vi "test Format RESP3.vi"() -> (0 "error out":errorcluster, 2 "pass?":bool)   [LabVIEW 2019, in "RESP3 Tests.lvlib"]
uses:
  RESP3 Tests.lvlib
  RESP3/RESP3 Parser/RESP3 Parser.lvclass
  RESP3/types/RESP3 data type attribute.vi
  RESP3/high-level/RESP3 Make Simple String.vi
  RESP3/high-level/RESP3 Make Simple Error.vi
  RESP3/high-level/RESP3 Make Bulk String.vi
  RESP3/high-level/RESP3 Make Bulk Error.vi
  RESP3/high-level/RESP3 Make Map.vi
  RESP3/high-level/RESP3 Make Attributes.vi
  RESP3/high-level/RESP3 Make Set.vi
  RESP3/high-level/RESP3 Make Array.vi
  RESP3/RESP3.lvlib
panel:
  out "values match?":bool
  out "RESP3 Value orig.":variant
  out "RESP3 Value reparsed":variant
  out "messages":string[](array[string])
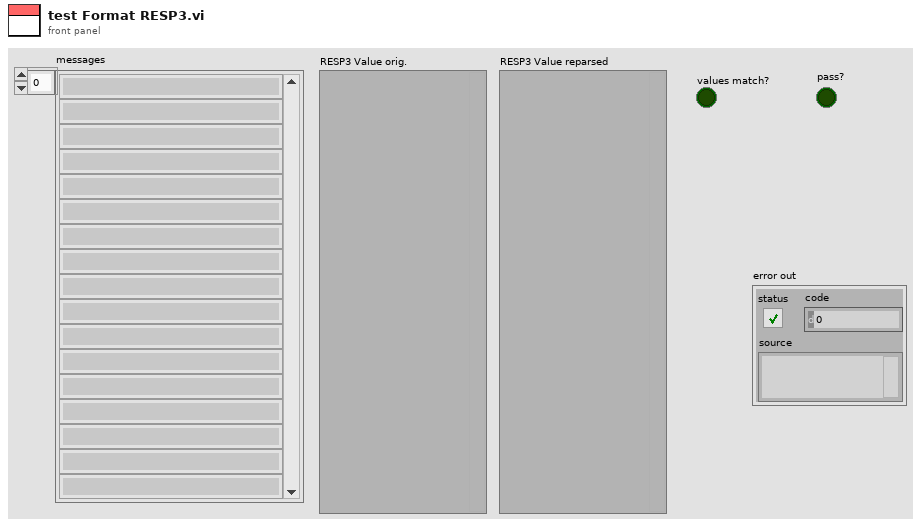
[diagram p1: front panel]
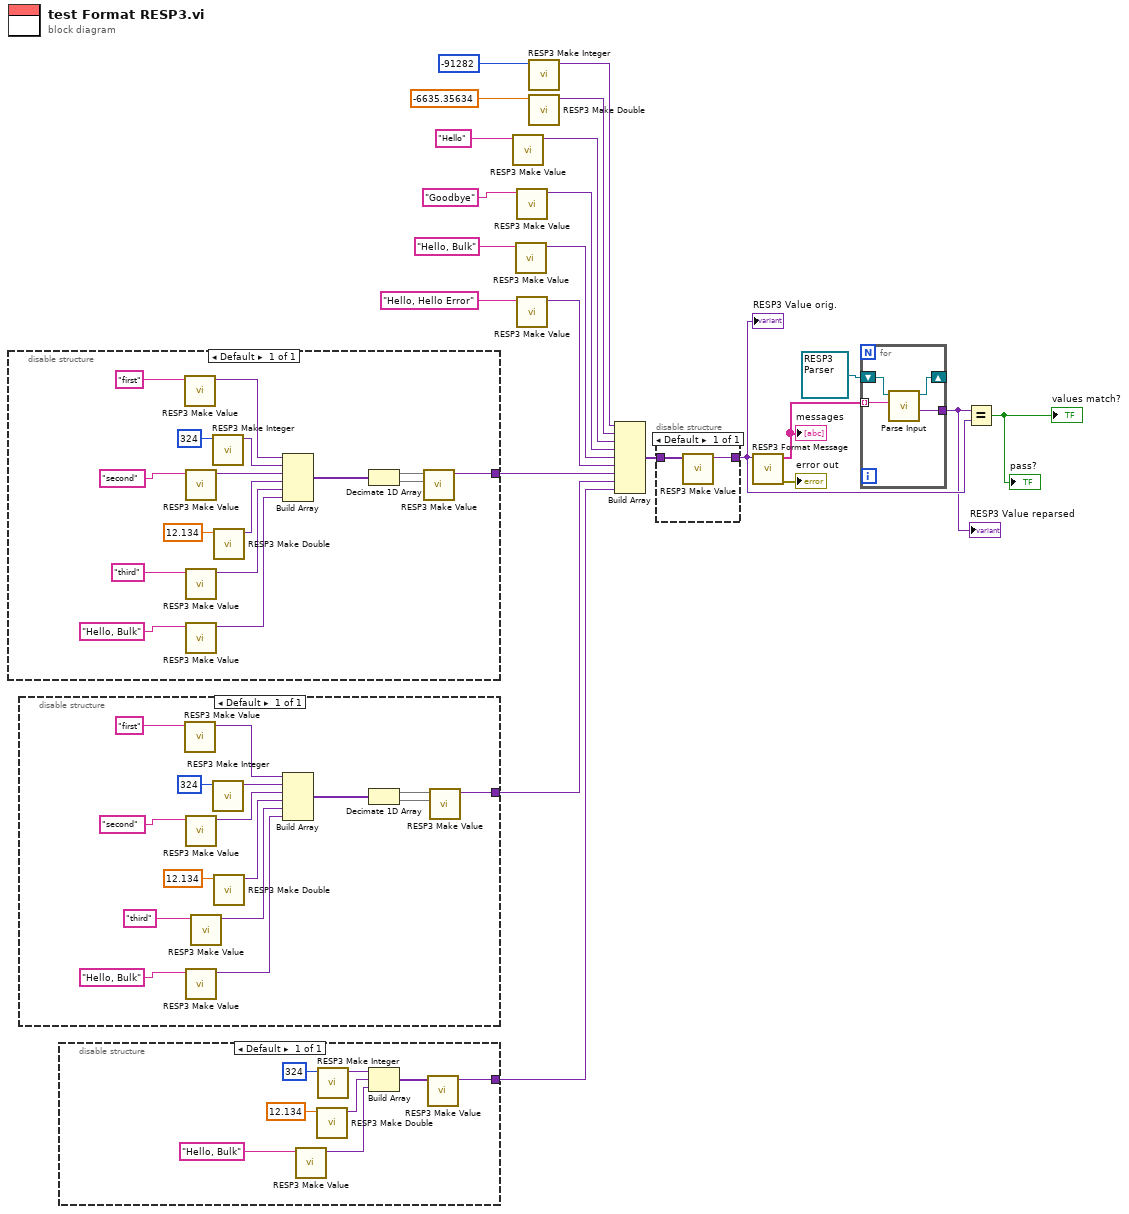
[diagram p0: block diagram]
diagram:
  n1 = disable-structure shown="Default" {
    disable-tunnel: [w26] -> w12
    frame Enabled {
      n2 = call-poly "RESP3 Make Value.vi"("String"="first" ("string in")) -> ("RESP3 Value out"=w37:variant)  [unwired: 9 in, 1 out]
      n3 = call-poly "RESP3 Make Value.vi"("String"="second" ("string in")) -> ("RESP3 Value out"=w35:variant)  [unwired: 9 in, 1 out]
      n4 = call-poly "RESP3 Make Value.vi"("String"="third" ("string in")) -> ("RESP3 Value out"=w33:variant)  [unwired: 9 in, 1 out]
      n5 = call-poly "RESP3 Make Value.vi"("String"="Hello, Bulk" ("string in")) -> ("RESP3 Value out"=w32:variant)  [unwired: 9 in, 1 out]
      n6 = call "RESP3 Make Integer.vi"("integer"=i64 324) -> ("RESP3 Value out"=w36:variant)  [unwired: 9 in, 1 out]
      n7 = call "RESP3 Make Double.vi"("double"=12.134) -> ("RESP3 Value out"=w34:variant)  [unwired: 9 in, 1 out]
      n8 = Build Array(w37, w36, w35, w34, w33, w32) -> (w25:variant[])
      n9 = Decimate 1D Array(w25) -> (w24:variant[], w23:variant[])
      n10 = call-poly "RESP3 Make Value.vi"("values (RESP3 values)"=w23, "keys (RESP3 values)"=w24) -> ("RESP3 Value out"=w26:variant)  [unwired: 8 in, 1 out]
    }
  }
  n11 = disable-structure shown="Default" {
    disable-tunnel: [w42] -> w5
    frame Enabled {
      n12 = call-poly "RESP3 Make Value.vi"("String"="first" ("string in")) -> ("RESP3 Value out"=w52:variant)  [unwired: 9 in, 1 out]
      n13 = call-poly "RESP3 Make Value.vi"("String"="second" ("string in")) -> ("RESP3 Value out"=w50:variant)  [unwired: 9 in, 1 out]
      n14 = call-poly "RESP3 Make Value.vi"("String"="Hello, Bulk" ("string in")) -> ("RESP3 Value out"=w47:variant)  [unwired: 9 in, 1 out]
      n15 = call-poly "RESP3 Make Value.vi"("String"="third" ("string in")) -> ("RESP3 Value out"=w48:variant)  [unwired: 9 in, 1 out]
      n16 = call "RESP3 Make Integer.vi"("integer"=i64 324) -> ("RESP3 Value out"=w51:variant)  [unwired: 9 in, 1 out]
      n17 = call "RESP3 Make Double.vi"("double"=12.134) -> ("RESP3 Value out"=w49:variant)  [unwired: 9 in, 1 out]
      n18 = Build Array(w52, w51, w50, w49, w48, w47) -> (w41:variant[])
      n19 = Decimate 1D Array(w41) -> (w40:variant[], w39:variant[])
      n20 = call-poly "RESP3 Make Value.vi"("values (RESP3 values)"=w39, "keys (RESP3 values)"=w40) -> ("RESP3 Value out"=w42:variant)  [unwired: 8 in, 1 out]
    }
  }
  n21 = disable-structure shown="Default" {
    disable-tunnel: [w56] -> w4
    frame Enabled {
      n22 = call-poly "RESP3 Make Value.vi"("String"="Hello, Bulk" ("string in")) -> ("RESP3 Value out"=w58:variant)  [unwired: 9 in, 1 out]
      n23 = call "RESP3 Make Double.vi"("double"=12.134) -> ("RESP3 Value out"=w59:variant)  [unwired: 9 in, 1 out]
      n24 = call "RESP3 Make Integer.vi"("integer"=i64 324) -> ("RESP3 Value out"=w60:variant)  [unwired: 9 in, 1 out]
      n25 = Build Array(w60, w59, w58) -> (w55:variant[])
      n26 = call-poly "RESP3 Make Value.vi"("RESP3 Values in"=w55) -> ("RESP3 Value out"=w56:variant)  [unwired: 9 in, 1 out]
    }
  }
  n27 = call-poly "RESP3 Make Value.vi"("String"="Hello" ("string in")) -> ("RESP3 Value out"=w17:variant)  [unwired: 9 in, 1 out]
  n28 = call-poly "RESP3 Make Value.vi"("String"="Hello, Bulk" ("string in")) -> ("RESP3 Value out"=w15:variant)  [unwired: 9 in, 1 out]
  n29 = call-poly "RESP3 Make Value.vi"("String"="Goodbye" ("string in")) -> ("RESP3 Value out"=w16:variant)  [unwired: 9 in, 1 out]
  n30 = call-poly "RESP3 Make Value.vi"("String"="Hello, Hello Error" ("string in")) -> ("RESP3 Value out"=w14:variant)  [unwired: 9 in, 1 out]
  n31 = call "RESP3 Make Integer.vi"("integer"=i64 -91282) -> ("RESP3 Value out"=w19:variant)  [unwired: 9 in, 1 out]
  n32 = call "RESP3 Make Double.vi"("double"=-6635.35634) -> ("RESP3 Value out"=w18:variant)  [unwired: 9 in, 1 out]
  n33 = Build Array(w19, w18, w17, w16, w15, w14, w12, w5, w4) -> (w7:variant[])
  n34 = disable-structure shown="Default" {
    disable-tunnel: w7 -> [w64]
    disable-tunnel: [w63] -> w9
    frame Enabled {
      n35 = call-poly "RESP3 Make Value.vi"("RESP3 Values in"=w64) -> ("RESP3 Value out"=w63:variant)  [unwired: 9 in, 1 out]
    }
  }
  "RESP3 Value orig." <- w9
  n36 = call "RESP3 Format Message.vi"("RESP3 Value"=w9) -> ("error out"=→"error out":errorcluster, "messages"=w11:string[])  [unwired: 9 in]
  "messages" <- w11
  n37 = for {
    tunnel: w11 -> [w67] mode=indexing
    shift-right: [w65] -> _
    shift-left: refnum<class "RESP3 Parser.lvclass"> refnum ("RESP3.lvlib:RESP3 Parser.lvclass") -> [w68]
    tunnel: [w66] -> w8
    n38 = call-dynamic "Parse Input.vi"("input line"=w67, "RESP3 Parser in"=w68) -> ("RESP3 Value"=w66:variant, "RESP3 Parser out"=w65:refnum<class "RESP3 Parser.lvclass">)  [unwired: 5 in, 3 out]
  }
  "RESP3 Value reparsed" <- w8
  n39 = Equal?(x=w8, y=w9) -> (x = y?=→"pass?" →"values match?":bool)
